vi "Configure Protection.vi"(6 "Protection (None)":T1, 8 "error in (no error)":errorcluster, 10 "Limit":dbl, 11 "2230G in":refnum<class "2230G.lvclass">) -> (0 "error out":errorcluster, 3 "2230G out":refnum<class "2230G.lvclass">)   [LabVIEW 2018, in "2230G.lvlib" / "2230G.lvclass"]
doc: "Configure Protection setting, available options:\n\n0: None\n1: Over Voltage\n2: Under Voltage\n3: Over Current\n\nDbl Precision Limit"
uses:
  2230G.lvclass
  PPLs/Power Supply/Parent/Power_Supply.lvlibp/Custom Control/Protection.ctl
  PPLs/Power Supply/Parent/Power_Supply.lvlibp/Power Supply.lvclass
  <instrlib>/Keithley KE22xx Series/Keithley KE22xx Series.lvlib
  C:/Projects/LabVIEW/PPLs/Power Supply/Parent/Power_Supply.lvlibp/Power Supply.lvclass
  PPLs/Power Supply/Parent/Power_Supply.lvlibp
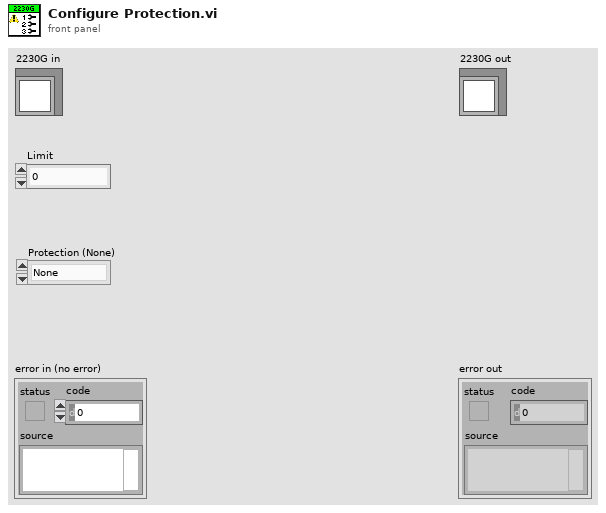
[diagram p1: front panel]
types:
  T1 = typedef "Power_Supply.lvlibp/Protection.ctl" = enum16{"None", "Over Volt", "Under Volt", "Over Current"}
  T2 = typedef "Power_Supply.lvlibp/Channel List.ctl" = enum16{"Channel 1", "Channel 2", "Channel 3", "Channel 4"}
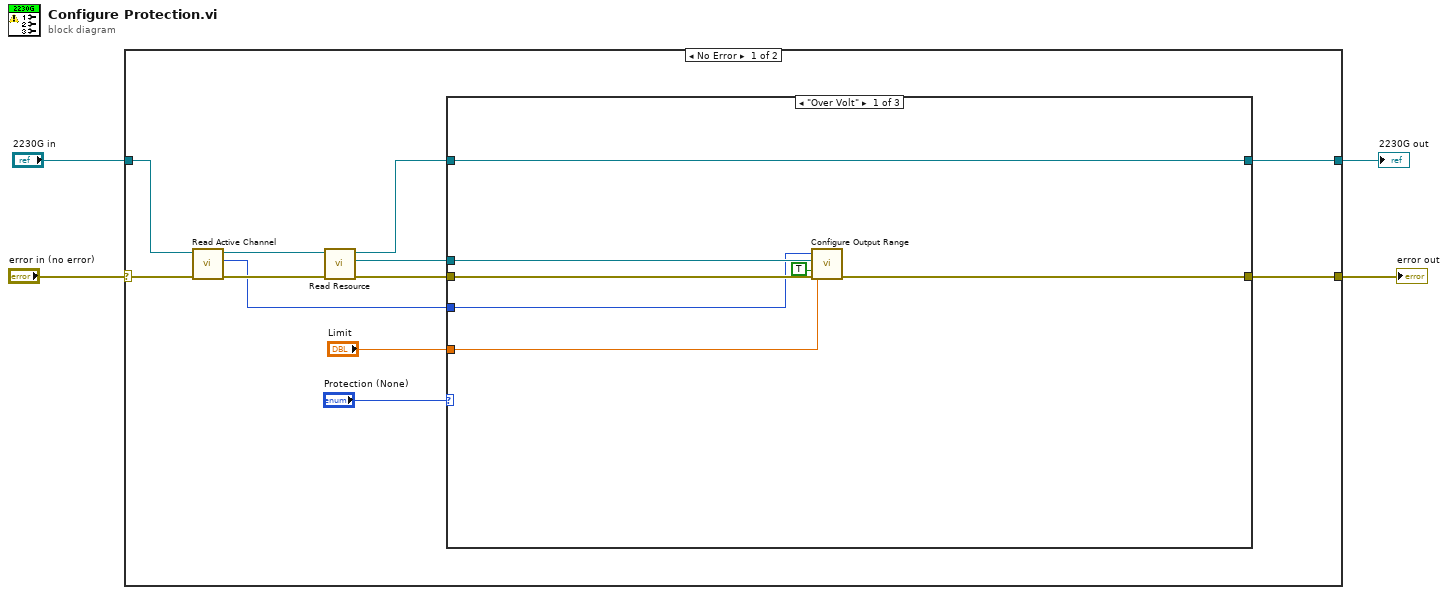
[diagram p0: block diagram]
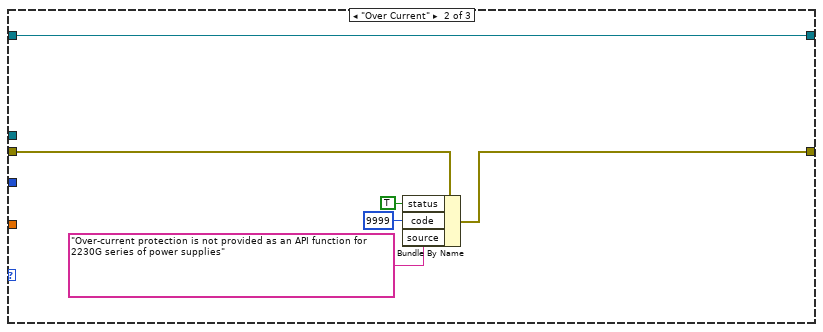
[diagram p2: hidden frame]
diagram:
  n1 = case shown="No Error" "error in (no error)" {
    selector: "error in (no error)" -> [w8 w33]
    tunnel: [w10 w33] -> w3
    tunnel: [w11 w32] -> w2
    tunnel: "2230G in" -> [w9 w32]
    frame No Error {
      n2 = call "Read Active Channel.vi"("error in (no error)"=w8, "Power Supply in"=w9) -> ("error out"=w7:errorcluster, "Active Channel"=w5:T2, "Power Supply out"=w6:refnum<class "2230G.lvclass">)  [unwired: 7 in]
      n3 = call "Read Resource.vi"("error in"=w7, "Power Supply in"=w6) -> ("error out"=w15:errorcluster, "Resource"=w14:refnum<visa-resource-name>, "Power Supply out"=w13:refnum<class "2230G.lvclass">)  [unwired: 7 in]
      n4 = case shown="\"Over Volt\"" "Protection (None)" {
        tunnel: w15 -> [w22 w28 w30]
        tunnel: w14 -> [w23 _ _]
        tunnel: w13 -> [w17 w29 w31]
        tunnel: "Limit" -> [w19 _ _]
        tunnel: [w17 w29 w31] -> w11
        tunnel: [w18 w24 w30] -> w10
        tunnel: w5 -> [w21 _ _]
        frame "Over Volt" {
          n5 = call <instrlib>:"Configure Output Range.vi"("VISA resource name"=w23, "Channel Select"=w21, "MAX Voltage Limit"=w19, "Enable Max. Voltage (T: Enable)"=TRUE, "error in (no error)"=w22) -> ("error out"=w18:errorcluster)  [unwired: 9 in, 1 out]
        }
        frame "Over Current" {
          n6 = Bundle By Name(cluster=w28, "status"=TRUE, "code"=9999, "source"="Over-current protection is not provided as an API function for 2230G series of power supplies") -> (w24:errorcluster)
        }
        frame Default {
        }
      }
    }
    frame Error {
    }
  }
  "error out" <- w3
  "2230G out" <- w2
